vi "Launcher.vi"   [LabVIEW 2023, in "Example Iterator NR Actor Implicit Iteration.lvlib"]
doc: "Launches the Example Actor that shows the operation of the Iterator Actor framework."
uses:
  Example Iterator NR Actor Implicit Iteration.lvlib
  <vilib>/ActorFramework/Actor/Actor.lvclass
  Example Actor/Example Actor.lvclass
panel:
  # "Launch this VI to start the example"
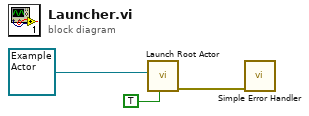
[diagram p0: block diagram]
diagram:
  n1 = call <vilib>:"Launch Root Actor.vi"("Open Actor Core front panel? (F)"=TRUE, "Actor"=refnum<class "Example Actor.lvclass"> refnum ("Example Iterator NR Actor.lvlib:Example Actor.lvclass")) -> ("error out"=w2:errorcluster)  [unwired: 8 in, 1 out]
  n2 = call <vilib>:"Simple Error Handler.vi"("error in (no error)"=w2) -> ()  [unwired: 4 in, 5 out]
